vi "TX-BPCS-SIM-Wired (SubVI).vi"(9 "BPCS-10AY300":dbl, 10 "BPCS-10TY100":dbl format="%.2f", 11 "BPCS-10Y200":dbl format="%.2f") -> (3 "BPCS-SIM-TX-ARRAY":dbl[](array[numeric]))   [LabVIEW 2018]
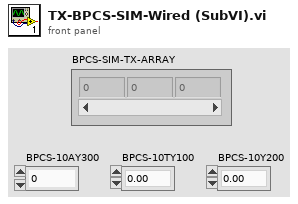
[diagram p1: front panel]
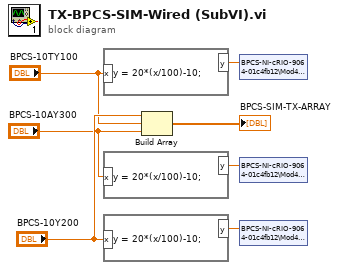
[diagram p0: block diagram]
diagram:
  n1 = formula code="y = 20*(x/100)-10;"("x"="BPCS-10TY100") -> ("y"=w6:dbl)
  n2 = formula code="y = 20*(x/100)-10;"("x"="BPCS-10AY300") -> ("y"=w5:dbl)
  n3 = formula code="y = 20*(x/100)-10;"("x"="BPCS-10Y200") -> ("y"=w7:dbl)
  n4 = Build Array("BPCS-10Y200", "BPCS-10TY100", "BPCS-10AY300") -> (→"BPCS-SIM-TX-ARRAY":dbl[])
  n5 = shared-variable "BPCS-NI-cRIO-9064-01c4fb12\\Mod4\\AO1"(w6) -> ()  [unwired: 1 in, 1 out]
  n6 = shared-variable "BPCS-NI-cRIO-9064-01c4fb12\\Mod4\\AO2"(w5) -> ()  [unwired: 1 in, 1 out]
  n7 = shared-variable "BPCS-NI-cRIO-9064-01c4fb12\\Mod4\\AO0"(w7) -> ()  [unwired: 1 in, 1 out]
